vi "TWM Parse Parameters.vi"(8 "error in (no error)":errorcluster, 11 "twm params":refnum<vi>) -> (0 "error out":errorcluster, 3 "parameters":T1[](array[typedef]))   [LabVIEW 2013]
uses:
  TWM parameters.ctl
  <vilib>/regexp/Match Regular Expression.xnode
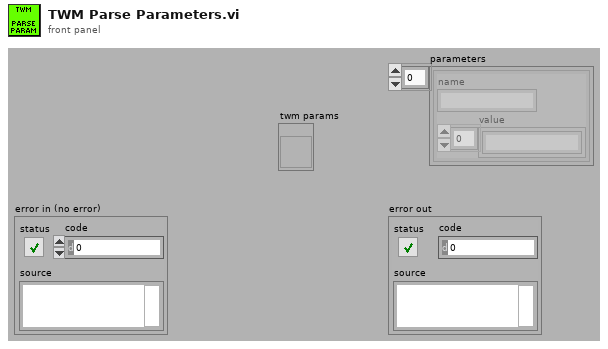
[diagram p1: front panel]
types:
  T1 = typedef "TWM parameters.ctl" = cluster{"name":string, "value":string[]}
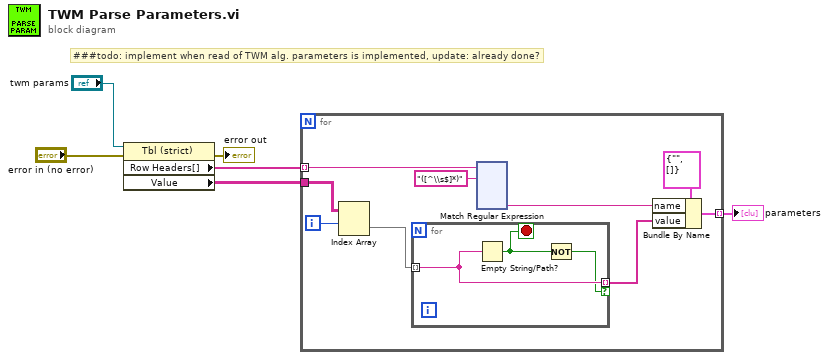
[diagram p0: block diagram]
diagram:
  # "###todo: implement when read of TWM alg. parameters is implemented, update: already done?"
  n1 = property class="Tbl (strict)"(reference="twm params", error in="error in (no error)") -> (error out=→"error out":errorcluster, "Row Headers[]"=w5:string[], "Value"=w4:string[][])  [unwired: 1 out]
  n2 = for {
    tunnel: w5 -> [w15] mode=indexing
    tunnel: w4 -> [w11]
    tunnel: [w12] -> w3 mode=indexing
    i -> [w10]
    n3 = Index Array(array=w11, index (row)=w10) -> (element=w9:string[])  [unwired: 1 in]
    n4 = for {
      tunnel: w9 -> [w18] mode=indexing
      tunnel: [w18] -> w7 mode=indexing if=w16
      stop <- w17 stop-if-true
      n5 = Empty String/Path?(string/path=w18) -> (empty?=w17:bool)
      n6 = Not(x=w17) -> (.not. x?=w16:bool)
    }
    n7 = xnode "Match Regular Expression"("input string"=w15, "regular expression"="([^\\s$]*)") -> ("submatch 1"=w13:string)  [unwired: 4 in, 5 out]
    n8 = Bundle By Name(cluster=T1 {"name"="", "value"=[]} ("parameters"), "name"=w13, "value"=w7) -> (w12:T1)
  }
  "parameters" <- w3
